vi "initialize.vi"(8 "error in (no error)":errorcluster, 11 "sequencer name":string) -> (0 "error out":errorcluster, 3 "Simple Sequencer API out":refnum<class "Simple Sequencer API.lvclass">)   [LabVIEW 2014, in "Simple Sequencer API.lvclass"]
doc: "Opens a session to a sequencer module running in an Engine identified by its 'sequencer name'."
uses:
  Simple Sequencer API.lvclass
  Simple Sequencer API.lvclass/Simple Sequencer API.ctl
  module/execution/Simple Sequencer TBM runtime.lvclass
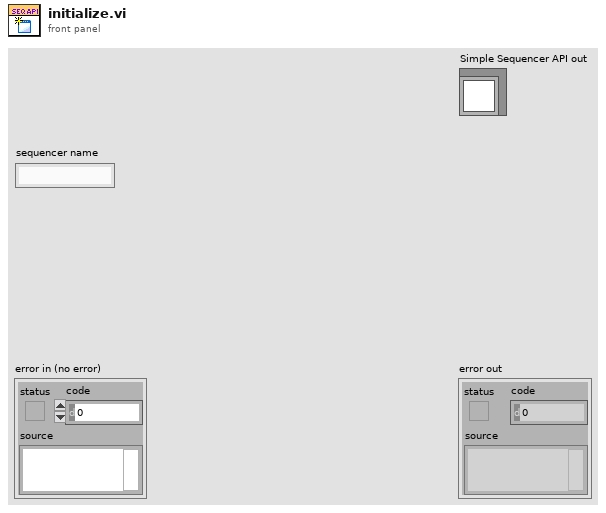
[diagram p1: front panel]
types:
  T1 = typedef "AMC.lvlib/Message Queue.ctl" = refnum<queue>
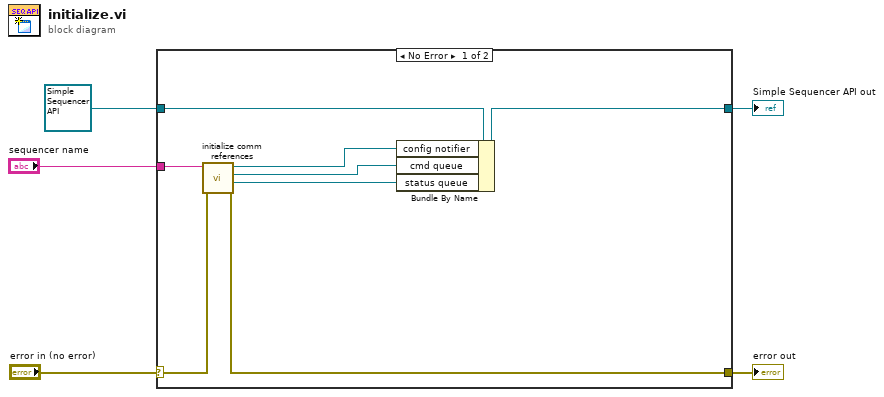
[diagram p0: block diagram]
diagram:
  n1 = case shown="No Error" "error in (no error)" {
    selector: "error in (no error)" -> [w12 w15]
    tunnel: [w11 w15] -> w4
    tunnel: [w6 w14] -> w3
    tunnel: refnum<class "Simple Sequencer API.lvclass"> refnum ("Simple Sequencer API in") -> [w10 w14]
    tunnel: "sequencer name" -> [w13 _]
    frame No Error {
      n2 = call "initialize comm references.vi"("error in (no error)"=w12, "sequencer name"=w13) -> ("error out"=w11:errorcluster, "message queue out"=w7:T1, "cmd queue out"=w8:T1, "config notifier out"=w9:refnum<notifier>)  [unwired: 6 in]
      n3 = Bundle By Name(cluster=w10, "config notifier"=w9, "cmd queue"=w8, "status queue"=w7) -> (w6:refnum<class "Simple Sequencer API.lvclass">)
    }
    frame Error {
    }
  }
  "error out" <- w4
  "Simple Sequencer API out" <- w3
